vi "Get Final Document Info.vi"(8 "error in":errorcluster, 11 "Lv Proj Document Type:TAF Proj":refnum<class "TAF Proj.lvclass">) -> (0 "error out":errorcluster, 2 "Final Documentation Info":T1)   [LabVIEW 2021, in "TAF Proj Document Type.lvlib" / "TAF Proj.lvclass"]
uses:
  <vilib>/Wovalab/AntiDoc/Document Type/Add-ons/LabVIEW TAF Project/TAF Proj/TAF Proj.lvclass
  C:/Program Files (x86)/National Instruments/LabVIEW 2021/vi.lib/Wovalab/AntiDoc/Document Type/Document/Document Type.lvclass
  <vilib>/Wovalab/AntiDoc/Document Type/Document/Final Documentation Info--cluster.ctl
  <vilib>/Wovalab/AntiDoc/Document Type/Add-ons/LabVIEW TAF Project/TAF Proj Config/TAF Proj Config.lvclass
  <vilib>/Wovalab/AntiDoc/Document Type/Document/Document Type.lvclass/Document Type.ctl
  <vilib>/Wovalab/AntiDoc/Document Type/Add-ons/LabVIEW TAF Project/TAF Proj Config/TAF Proj Config.lvclass/TAF Proj Config.ctl
  <vilib>/Wovalab/AntiDoc/Document Type/Document/Read Config.vi
  <vilib>/Wovalab/AntiDoc/Document Type/Add-ons/LabVIEW TAF Project/TAF Proj Config/Read Document Title.vi
  <vilib>/Wovalab/AntiDoc/Document Type/Add-ons/LabVIEW TAF Project/TAF Proj Config/Read Author.vi
  <vilib>/Wovalab/AntiDoc/Document Type/Add-ons/LabVIEW TAF Project/TAF Proj Config/Read E-mail.vi
  <vilib>/Wovalab/AntiDoc/Document Type/Add-ons/LabVIEW TAF Project/TAF Proj Config/Read Project Path.vi
  <vilib>/Wovalab/AntiDoc/Document Type/Config/Config.lvclass
  <vilib>/Wovalab/AntiDoc/Document Type/Document/Document Type.lvclass
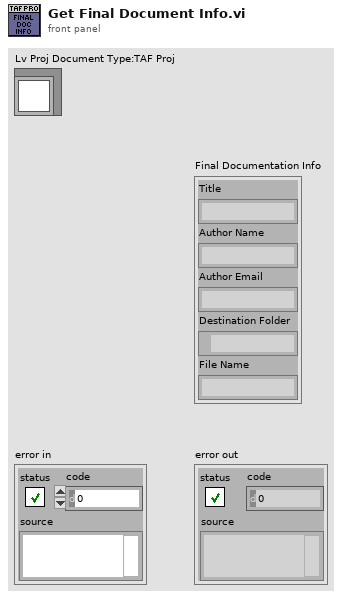
[diagram p1: front panel]
types:
  T1 = typedef "AntiDoc.lvlib/Document Type.lvclass/Final Documentation Info--cluster.ctl" = cluster{"Title":string, "Author Name":string, "Author Email":string, "Destination Folder":path, "File Name":string}
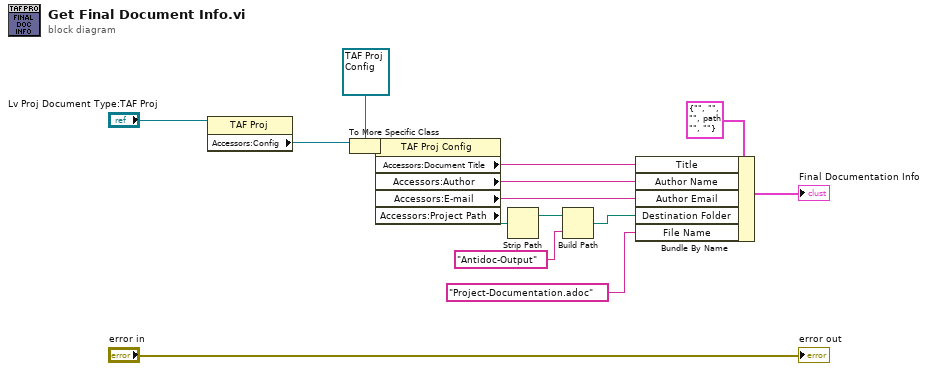
[diagram p0: block diagram]
diagram:
  n1 = property class="TAF Proj"(reference="Lv Proj Document Type:TAF Proj") -> ("Accessors:Config"=w13:refnum<class "Config.lvclass">)  [unwired: 1 in, 2 out]
  n2 = To More Specific Class(target class=refnum<class "TAF Proj Config.lvclass"> refnum ("Lv Proj Document Type.lvlib:Config"), reference=w13) -> (specific class reference=w11:refnum<class "TAF Proj Config.lvclass">)  [unwired: 1 in, 1 out]
  n3 = property class="TAF Proj Config"(reference=w11) -> ("Accessors:Document Title"=w4:string, "Accessors:Author"=w3:string, "Accessors:E-mail"=w2:string, "Accessors:Project Path"=w8:path)  [unwired: 1 in, 2 out]
  n4 = Strip Path(path=w8) -> (stripped path=w9:path)  [unwired: 1 out]
  n5 = Build Path(base path=w9, name or relative path="Antidoc-Output") -> (appended path=w6:path)
  n6 = Bundle By Name(cluster=T1 {"Title"="", "Author Name"="", "Author Email"="", "Destination Folder"=path "", "File Name"=""} ("Final Documentation Info"), "Title"=w4, "Author Name"=w3, "Author Email"=w2, "Destination Folder"=w6, "File Name"="Project-Documentation.adoc" ("name or relative path")) -> (→"Final Documentation Info":T1)
  "error out" <- "error in"
